vi "Get Angle Errors.vi"(2 "Offsets":T4, 3 "Kinematics Data":T1, 4 "Encoder Data":T5) -> (0 "Angle Errors":T2, 1 "Drive Powers":T3)   [LabVIEW 2018]
uses:
  Encoder Data.ctl
  Motor Data.ctl
  Error Data.ctl
  Kinematics Data.ctl
  <vilib>/Rock Robotics/Network Tables/NT Write Number.vi
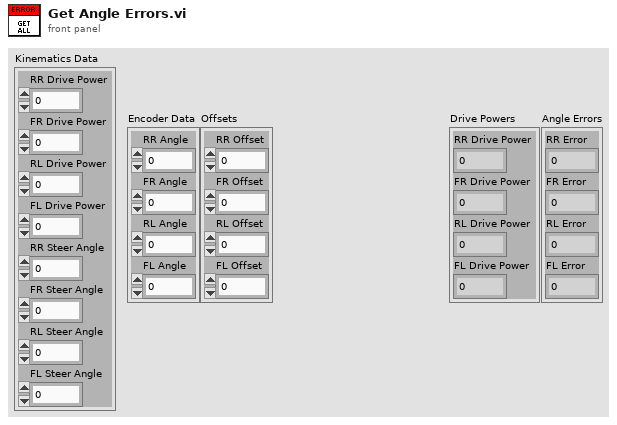
[diagram p1: front panel]
types:
  T1 = typedef "Kinematics Data.ctl" = cluster{"RR Drive Power":dbl, "FR Drive Power":dbl, "RL Drive Power":dbl, "FL Drive Power":dbl, "RR Steer Angle":dbl, "FR Steer Angle":dbl, "RL Steer Angle":dbl, "FL Steer Angle":dbl}
  T2 = typedef "Error Data.ctl" = cluster{"RR Error":dbl, "FR Error":dbl, "RL Error":dbl, "FL Error":dbl}
  T3 = typedef "Motor Data.ctl" = cluster{"RR Drive Power":dbl, "FR Drive Power":dbl, "RL Drive Power":dbl, "FL Drive Power":dbl}
  T4 = cluster{"RR Offset":dbl, "FR Offset":dbl, "RL Offset":dbl, "FL Offset":dbl}
  T5 = typedef "Encoder Data.ctl" = cluster{"RR Angle":dbl, "FR Angle":dbl, "RL Angle":dbl, "FL Angle":dbl}
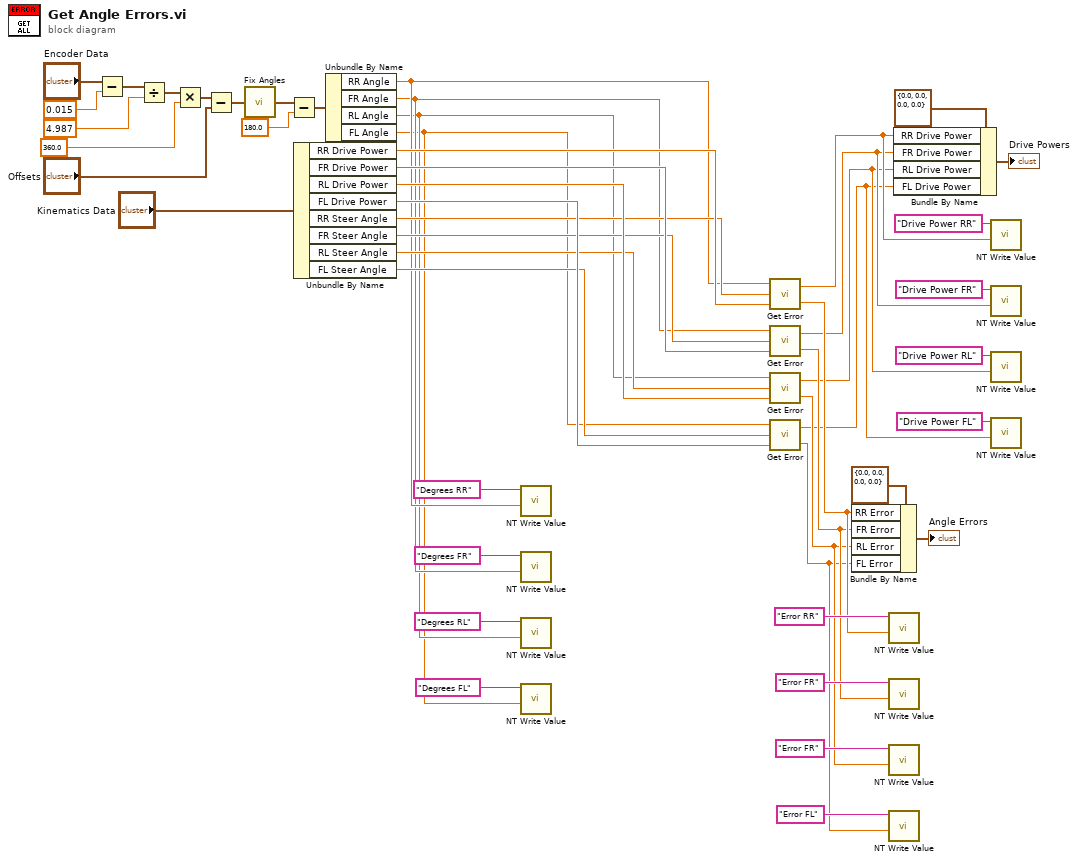
[diagram p0: block diagram]
diagram:
  n1 = Subtract(x="Encoder Data", y=0.015) -> (x-y=w47:T5)
  n2 = Divide(x=w47, y=4.987) -> (x/y=w45:T5)
  n3 = Multiply(x=w45, y=360.0) -> (x*y=w43:T5)
  n4 = Subtract(x=w43, y="Offsets") -> (x-y=w41:T5)
  n5 = call "Fix Angles.vi"("Input Angles"=w41) -> ("Output Angles"=w40:T5)
  n6 = Subtract(x=w40, y=180.0) -> (x-y=w38:T5)
  n7 = Unbundle By Name("Kinematics Data") -> ("RR Drive Power"=w32:dbl, "FR Drive Power"=w31:dbl, "RL Drive Power"=w30:dbl, "FL Drive Power"=w29:dbl, "RR Steer Angle"=w28:dbl, "FR Steer Angle"=w27:dbl, "RL Steer Angle"=w26:dbl, "FL Steer Angle"=w25:dbl)
  n8 = Unbundle By Name(w38) -> ("RR Angle"=w24:dbl, "FR Angle"=w23:dbl, "RL Angle"=w22:dbl, "FL Angle"=w21:dbl)
  n9 = call-poly <vilib>:"NT Write Value.vi"("Numeric"=w24, "Name"="Degrees RR") -> ()  [unwired: 9 in, 1 out]
  n10 = call-poly <vilib>:"NT Write Value.vi"("Numeric"=w23, "Name"="Degrees FR") -> ()  [unwired: 9 in, 1 out]
  n11 = call-poly <vilib>:"NT Write Value.vi"("Numeric"=w22, "Name"="Degrees RL") -> ()  [unwired: 9 in, 1 out]
  n12 = call-poly <vilib>:"NT Write Value.vi"("Numeric"=w21, "Name"="Degrees FL") -> ()  [unwired: 9 in, 1 out]
  n13 = call "Get Error.vi"("Motor Power"=w32, "Desired Angle"=w28, "Actual Angle"=w24) -> ("Angle Error"=w12:dbl, "Motor Power"=w4:dbl)
  n14 = call "Get Error.vi"("Motor Power"=w31, "Desired Angle"=w27, "Actual Angle"=w23) -> ("Angle Error"=w11:dbl, "Motor Power"=w3:dbl)
  n15 = call "Get Error.vi"("Motor Power"=w30, "Desired Angle"=w26, "Actual Angle"=w22) -> ("Angle Error"=w10:dbl, "Motor Power"=w2:dbl)
  n16 = call "Get Error.vi"("Motor Power"=w29, "Desired Angle"=w25, "Actual Angle"=w21) -> ("Angle Error"=w9:dbl, "Motor Power"=w1:dbl)
  n17 = Bundle By Name(cluster=T2 {"RR Error"=0.0, "FR Error"=0.0, "RL Error"=0.0, "FL Error"=0.0} ("Cluster"), "RR Error"=w12, "FR Error"=w11, "RL Error"=w10, "FL Error"=w9) -> (→"Angle Errors":T2)
  n18 = call-poly <vilib>:"NT Write Value.vi"("Numeric"=w12, "Name"="Error RR") -> ()  [unwired: 9 in, 1 out]
  n19 = call-poly <vilib>:"NT Write Value.vi"("Numeric"=w11, "Name"="Error FR") -> ()  [unwired: 9 in, 1 out]
  n20 = call-poly <vilib>:"NT Write Value.vi"("Numeric"=w10, "Name"="Error FR") -> ()  [unwired: 9 in, 1 out]
  n21 = call-poly <vilib>:"NT Write Value.vi"("Numeric"=w9, "Name"="Error FL") -> ()  [unwired: 9 in, 1 out]
  n22 = Bundle By Name(cluster=T3 {"RR Drive Power"=0.0, "FR Drive Power"=0.0, "RL Drive Power"=0.0, "FL Drive Power"=0.0}, "RR Drive Power"=w4, "FR Drive Power"=w3, "RL Drive Power"=w2, "FL Drive Power"=w1) -> (→"Drive Powers":T3)
  n23 = call-poly <vilib>:"NT Write Value.vi"("Numeric"=w4, "Name"="Drive Power RR") -> ()  [unwired: 9 in, 1 out]
  n24 = call-poly <vilib>:"NT Write Value.vi"("Numeric"=w3, "Name"="Drive Power FR") -> ()  [unwired: 9 in, 1 out]
  n25 = call-poly <vilib>:"NT Write Value.vi"("Numeric"=w2, "Name"="Drive Power RL") -> ()  [unwired: 9 in, 1 out]
  n26 = call-poly <vilib>:"NT Write Value.vi"("Numeric"=w1, "Name"="Drive Power FL") -> ()  [unwired: 9 in, 1 out]
